vi "Formula_Node_Ejercicio.vi"() -> ()   [LabVIEW 2020]
panel:
  out "output cluster":cluster{"X":dbl, "Y":dbl}[](graph)
  out "Waveform Chart":dbl[](graph)
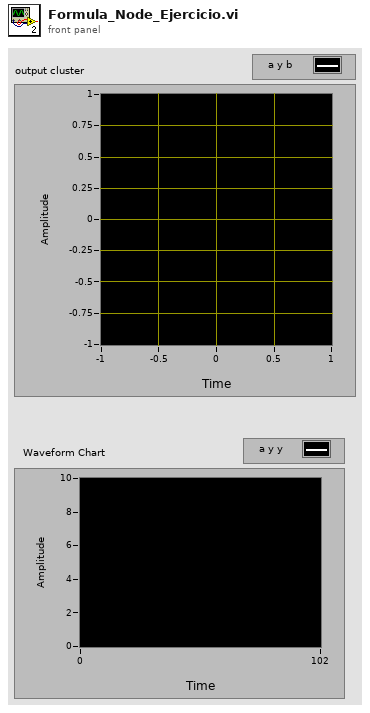
[diagram p1: front panel]
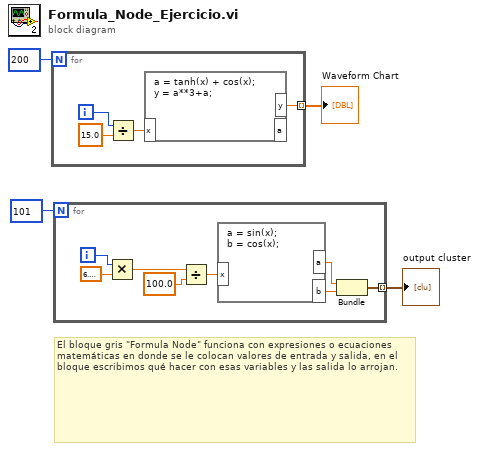
[diagram p0: block diagram]
diagram:
  # "El bloque gris \"Formula Node\" funciona con expresiones o ecuaciones matemáticas en donde se le colocan valores de entrada y salida, en el bloque escribimos qué hacer con esas variables y las salida lo arrojan."
  n1 = for {
    N: 200 -> [_]
    tunnel: [w5] -> w3 mode=indexing
    i -> [w6]
    n2 = Divide(x=w6, y=15.0) -> (x/y=w7:dbl)
    n3 = formula code="a = tanh(x) + cos(x);\ny = a**3+a;"("x"=w7) -> ("y"=w5:dbl)  [unwired: 1 out]
  }
  "Waveform Chart" <- w3
  n4 = for {
    N: 101 -> [_]
    tunnel: [w9] -> w1 mode=indexing
    i -> [w16]
    n5 = Multiply(x=w16, y=6.283185307179586) -> (x*y=w14:dbl)
    n6 = Divide(x=w14, y=100.0) -> (x/y=w12:dbl)
    n7 = formula code="a = sin(x);\nb = cos(x);"("x"=w12) -> ("a"=w11:dbl, "b"=w10:dbl)
    n8 = Bundle("a"=w11, "b"=w10) -> (w9:cluster{"a":dbl, "b":dbl})  [unwired: 1 in]
  }
  "output cluster" <- w1
